vi "labview_python_add_num.vi"() -> ()   [LabVIEW 2025]
panel:
  in  "python version":enum16{"3.6", "3.7", "3.8", "3.9", "3.10"}(ring)
  out "a+b":dbl
  in  "b":dbl
  in  "a":dbl
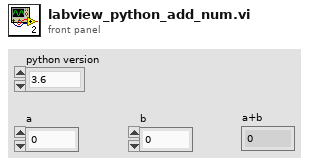
[diagram p1: front panel]
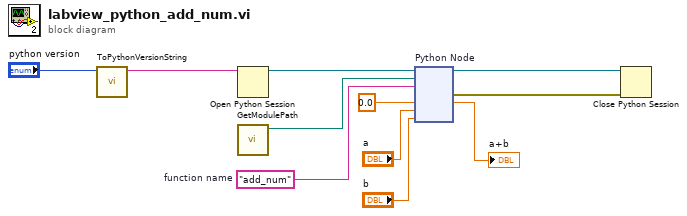
[diagram p0: block diagram]
diagram:
  w10 = "add_num"  # function name
  n1 = call "ToPythonVersionString.vi"("python version"="python version") -> ("python version string"=w1:string)  [unwired: 10 in]
  n2 = Open Python Session(python version=w1) -> (session out=w11:refnum<k35>)  [unwired: 2 in, 1 out]
  n3 = call "GetModulePath.vi"() -> ("module path"=w3:path)  [unwired: 11 in]
  n4 = node "Python Node"(w11, w3, w10, 0.0, "a", "b") -> (w5:refnum<k35>, w4:errorcluster, →"a+b":dbl)  [unwired: 3 in, 2 out]
  n5 = Close Python Session(session in=w5, error in=w4) -> ()  [unwired: 1 out]
